vi "GLOBAL_Dig1.vi"(4 "Data in":sgl[][](array[numeric]), 5 "State":enum16{"Initialise", "Write", "Read"}(ring)) -> (1 "Valid Read?":bool, 2 "Data Out":sgl[][](array[numeric]))   [LabVIEW 2014]
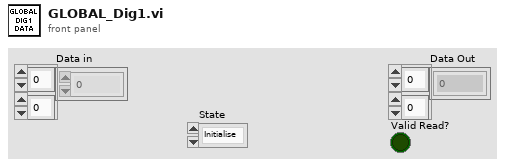
[diagram p1: front panel]
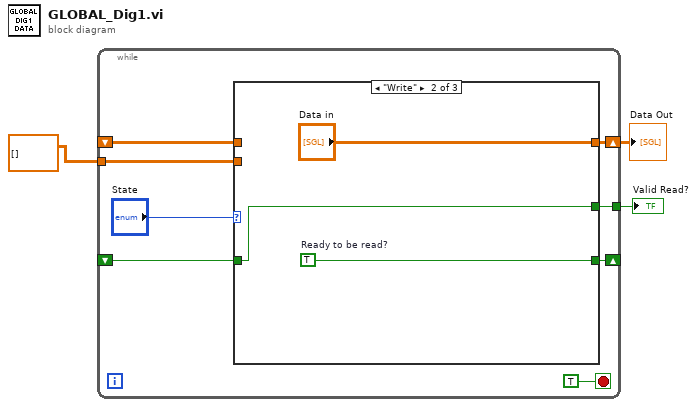
[diagram p0: block diagram]
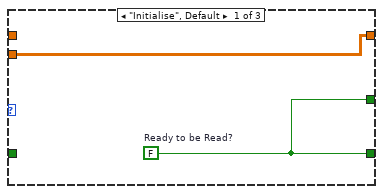
[diagram p2: hidden frame]
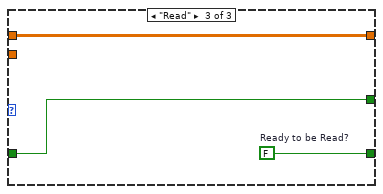
[diagram p3: hidden frame]
diagram:
  n1 = while {
    shift-right: [w10] -> w2
    shift-left: _ -> [w4]
    shift-right: [w8] -> _
    shift-left: _ -> [w7]
    tunnel: [w6] -> w1
    tunnel: sgl[][] [] ("Channel Data") -> [w5]
    stop <- TRUE stop-if-true
    n2 = case shown="\"Write\"" "State" {
      tunnel: [w12 "Data in" w18] -> w10
      tunnel: w4 -> [_ _ w18]
      tunnel: [w13 w16 w19] -> w8
      tunnel: w7 -> [_ w15 w17]
      tunnel: [w13 w15 w17] -> w6
      tunnel: w5 -> [w12 _ _]
      frame "Initialise", Default {
        w13 = FALSE  # Ready to be Read?
      }
      frame "Write" {
        w16 = TRUE  # Ready to be read?
      }
      frame "Read" {
        w19 = FALSE  # Ready to be Read?
      }
    }
  }
  "Data Out" <- w2
  "Valid Read?" <- w1
